vi "Instrumento virtual.vi"() -> ()   [LabVIEW 2020]
panel:
  out "LED ON time":dbl
  in  "Horizontal Pointer Slide":dbl(slide) scale=0.0..250.0
  in  "Current Box":u32(colorbox)
  out "Waveform Chart":dbl(graph)
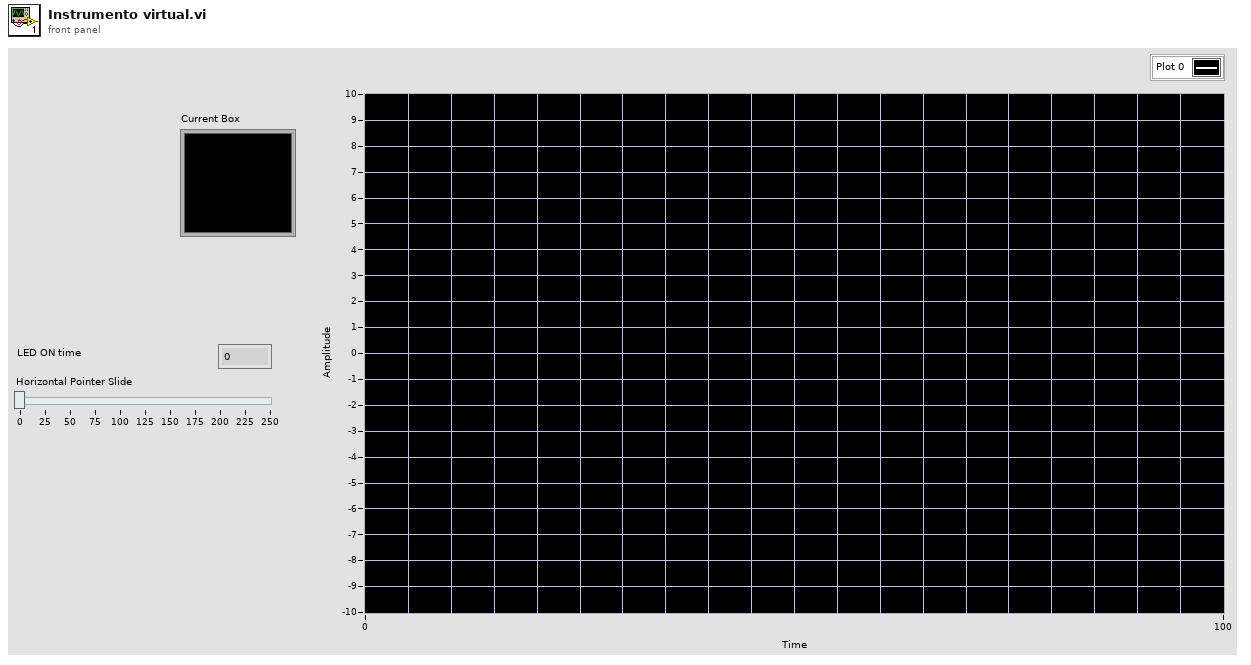
[diagram p1: front panel]
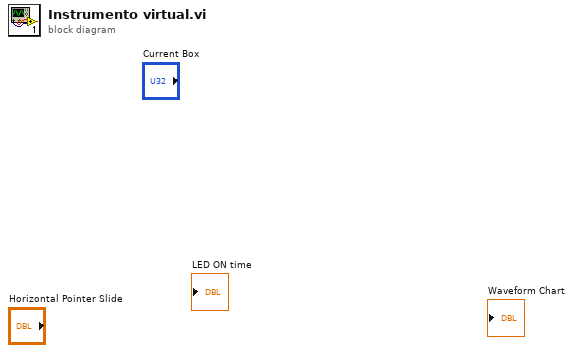
[diagram p0: block diagram]
diagram:
